vi "Create G-CLI Script quitLabVIEW.vi"(8 "error in (no error)":errorcluster, 11 "PostBuildSupport in":refnum<class "PostBuildSupport.lvclass">) -> (0 "error out":errorcluster, 2 "command":string, 3 "PostBuildSupport out":refnum<class "PostBuildSupport.lvclass">)   [LabVIEW 2019, in "PostBuildSupport.lvclass"]
uses:
  PostBuildSupport.lvclass
  PostBuildSupport.lvclass/PostBuildSupport.ctl
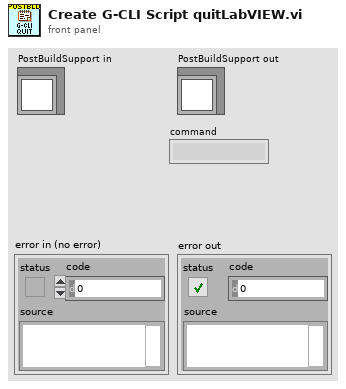
[diagram p1: front panel]
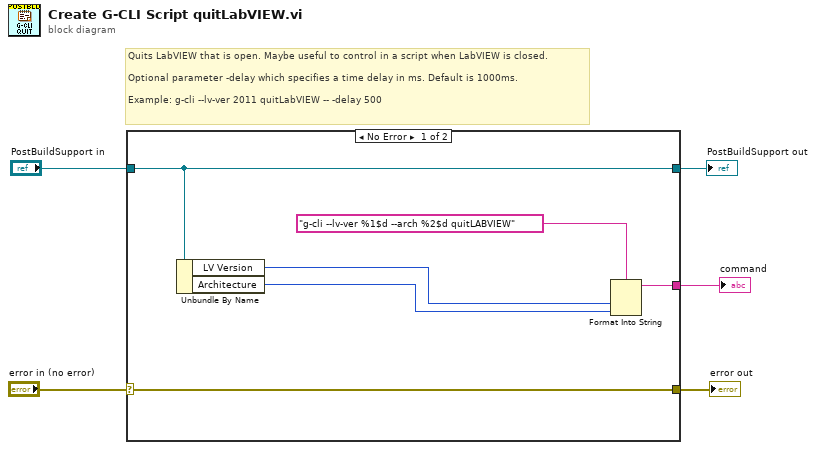
[diagram p0: block diagram]
diagram:
  # "Quits LabVIEW that is open. Maybe useful to control in a script when LabVIEW is closed.\n\nOptional parameter -delay which specifies a time delay in ms. Default is 1000ms.\n\nExample: g-cli --lv-ver 2011 quitLabVIEW -- -delay 500"
  n1 = case shown="No Error" "error in (no error)" {
    selector: "error in (no error)" -> [w6 w13]
    tunnel: "PostBuildSupport in" -> [w11 w12]
    tunnel: [w6 w13] -> w3
    tunnel: [w11 w12] -> w2
    tunnel: [w7 _] -> w1
    frame No Error {
      n2 = Unbundle By Name(w11) -> ("LV Version"=w9:u32, "Architecture"=w8:u32)
      n3 = Format Into String(format string="g-cli --lv-ver %1$d --arch %2$d quitLABVIEW", w9, w8) -> (resulting string=w7:string)  [unwired: 2 in, 1 out]
    }
    frame Error {
    }
  }
  "error out" <- w3
  "PostBuildSupport out" <- w2
  "command" <- w1
